vi "PhotonUtils_CalculateDistanceToTarget.vi"(8 "TargetPitch_Radians":dbl, 9 "CameraPitch_Radians":dbl, 10 "TargetHeight_Meters":dbl, 11 "CameraHeight_Meters":dbl) -> (3 "DistanceToTarget_Meters":dbl)   [LabVIEW 2019, in "PhotonVisionLib.lvlib"]
doc: "Algorithm from https://docs.limelightvision.io/en/latest/cs_estimating_distance.html Estimates range to a target using the target's elevation. This method can produce more stable results than SolvePNP when well tuned, if the full 6d robot pose is not required. Note that this method requires the camera to have 0 roll (not be skewed clockwise or CCW relative to the floor), and for there to exist a height differential between goal and camera. The larger this differential, the more accurate the distance estimate will be.\n \nUnits can be converted using the {@link edu.wpi.first.math.util.Units} class.\n \nInputs:\n - CameraHeight_Meters -- The physical height of the camera off the floor \n in meters.\n - TargetHeightMeters -- The physical height of the target off the floor in meters. \n This should be the height of whatever is being targeted (i.e. if the \n targeting region is set to top, this should be the height of the top \n of the target).\n - CameraPitch_Radians -- The pitch of the camera from the horizontal plane \n in radians.\n Positive values up.\n - TargetPitchRadian -- The pitch of the target in the camera's lens in radians. \n Positive values up.\n\nOutputs\n - DistanceToTarget_Meters -- The estimated distance to the target in meters."
uses:
  PhotonVisionLib.lvlib
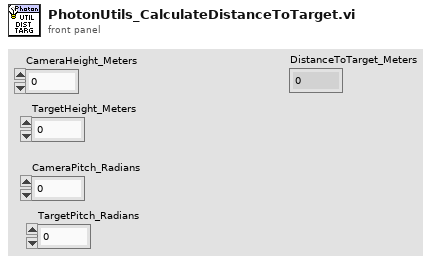
[diagram p1: front panel]
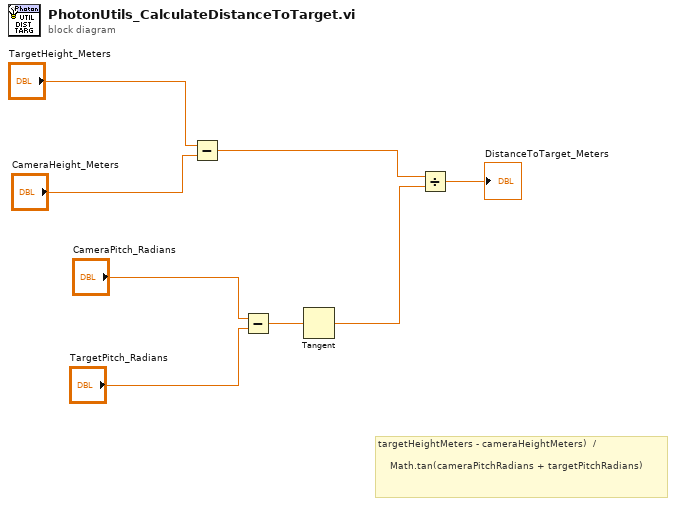
[diagram p0: block diagram]
diagram:
  # "targetHeightMeters - cameraHeightMeters)  /\n      \n    Math.tan(cameraPitchRadians + targetPitchRadians)"
  n1 = Subtract(x="TargetHeight_Meters", y="CameraHeight_Meters") -> (x-y=w3:dbl)
  n2 = Subtract(x="CameraPitch_Radians", y="TargetPitch_Radians") -> (x-y=w4:dbl)
  n3 = Tangent(1:w4) -> (0:w2:dbl)
  n4 = Divide(x=w3, y=w2) -> (x/y=→"DistanceToTarget_Meters":dbl)
